vi "Get Default Printer Name.vi"(2 "Error In":errorcluster) -> (0 "Error Out":errorcluster, 1 "Default Printer Name":string)   [LabVIEW 2016]
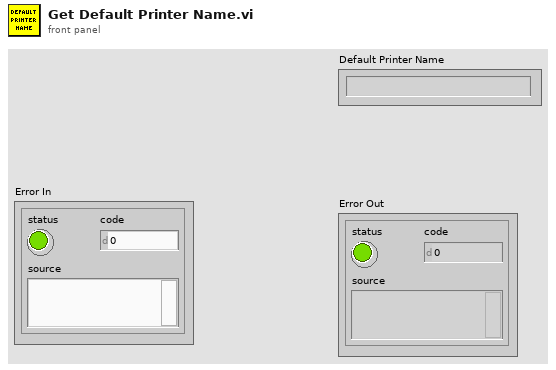
[diagram p1: front panel]
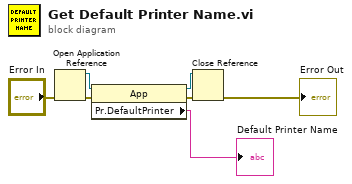
[diagram p0: block diagram]
diagram:
  n1 = Open Application Reference(8:"Error In") -> (0:w7:errorcluster, 3:w5:refnum<vi>)  [unwired: 3 in]
  n2 = property class="App"(reference=w5, error in=w7) -> (reference out=w6:refnum<vi>, error out=w4:errorcluster, "Pr.DefaultPrinter"=→"Default Printer Name":string)
  n3 = Close Reference(reference=w6, error in (no error)=w4) -> (error out=→"Error Out":errorcluster)
